vi "PH_AWG-510.PC Write PSDB.vi"(0 "i ref in":refnum<vi>, 5 "error IO":errorcluster) -> (14 "i ref out":refnum<vi>, 19 "error out":errorcluster)   [LabVIEW 2014, in "PH_AWG-510.lvlib"]
doc: "This is the proc case which writes data to the PHELIX shot data base."
uses:
  PH_AWG-510.lvlib
  PH_Basics/PH_PSDBWriter/PH_PSDBWriter.PSDB Dataset.ctl
  PH_Basics/PH_PSDBWriter/PH_PSDBWriter.2D dataset.ctl
  CSlibraries-extern/psdb_lv/PSDB_AxisDescription.ctl
  PH_Basics/PH_PSDBWriter/PH_PSDBWriter.Boolean dataset.ctl
  PH_Basics/PH_PSDBWriter/PH_PSDBWriter.Image dataset.ctl
  <vilib>/vision/Image Controls.llb/IMAQ Image.ctl
  PH_Basics/PH_PSDBWriter/PH_PSDBWriter.Numeric dataset.ctl
  PH_Basics/PH_PSDBWriter/PH_PSDBWriter.String dataset.ctl
  PH_Basics/PH_PSDBWriter/PH_PSDBWriter.lvlib
  CSlibraries-extern/psdb_lv/PSDB.lvlib
  PH_Basics/PH_StatusHandler/PH_StatusHandler.lvlib
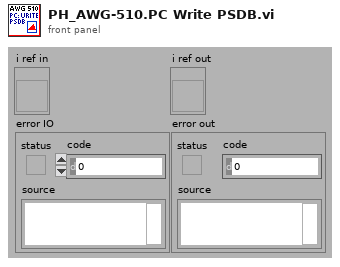
[diagram p1: front panel]
types:
  T1 = typedef "PH_PSDBWriter.lvlib/PH_PSDBWriter.PSDB Dataset.ctl" = cluster{"Version":i32, "2D data Input":T2[], "Boolean Input":T4[], "Image Input":T5[], "Numeric Input":T7[], "String Input":T8[]}
  T2 = typedef "PH_PSDBWriter.lvlib/PH_PSDBWriter.2D dataset.ctl" = cluster{"name":string, "data":dbl[][], "axis description":T3}
  T3 = typedef "PSDB.lvlib/PSDB_AxisDescription.ctl" = cluster{"x axis label":string, "y axis label":string, "x axis unit":string, "y axis unit":string}
  T4 = typedef "PH_PSDBWriter.lvlib/PH_PSDBWriter.Boolean dataset.ctl" = cluster{"name":string, "data":bool, "unit":string}
  T5 = typedef "PH_PSDBWriter.lvlib/PH_PSDBWriter.Image dataset.ctl" = cluster{"name":string, "data":T6, "unit":string}
  T6 = typedef "IMAQ Image.ctl" = refnum<image>
  T7 = typedef "PH_PSDBWriter.lvlib/PH_PSDBWriter.Numeric dataset.ctl" = cluster{"name":string, "data":dbl, "unit":string}
  T8 = typedef "PH_PSDBWriter.lvlib/PH_PSDBWriter.String dataset.ctl" = cluster{"name":string, "data":string, "unit":string}
  T9 = typedef "PH_AWG-510.lvlib/PH_AWG-510.i attribute.ctl" = cluster{"GUI Refs":cluster{"Delete":refnum<vi>, "Trigger Settings":refnum<vi>, "Start Device":refnum<vi>, "Instrument Information":refnum<vi>, "Lock Frontpanel":refnum<vi>, "Waveform Pattern File":refnum<vi>, "Initialize":refnum<vi>, "Output Settings":refnum<vi>}, "Instrument Information":T10, "Initialized?":bool, "Current Settings":cluster{"Trigger":T11, "Output Settings":T12}, "Wanted Settings":cluster{"Trigger":T11, "Output Settings":T12}, "Device frontpanel locked?":bool, "Default File Path":path}
  T10 = typedef "PH_AWG-510.lvlib/PH_AWG-510.Instrument Information Dataset.ctl" = cluster{"VISA resource name":refnum<visa-resource-name>, "Instrument Firmware Revision":string, "Manufacturer":string, "Model":string, "Serial Number":string, "Error Message":string, "Device Status":enum16{"stopped", "wating for trigger", "running", "Failure"}}
  T11 = typedef "PH_AWG-510.lvlib/PH_AWG-510.Trigger Settings.ctl" = cluster{"Mode":enum16{"Continuous", "Triggered", "Gated", "Enhanced"}, "Level (V)":dbl, "External Source":bool}
  T12 = typedef "PH_AWG-510.lvlib/PH_AWG-510.Output Settings.ctl" = cluster{"Activate Channel":bool, "VPP (V)":dbl, "Clock (Hz)":dbl, "File Name (Device)":string, "#1":u16, "#2":u16, "#3":u16, "#4":u16, "#5":u16, "#6":u16, "#7":u16, "#8":u16, "#9":u16, "#10":u16, "#11":u16, "#12":u16, "#13":u16, "#14":u16, "#15":u16, "#16":u16, "#17":u16, "#18":u16, "#19":u16, "#20":u16, "Offset (V)":dbl}
  T13 = typedef "PH_StatusHandler.lvlib/PH_StatusHandler.Status.ctl" = i16
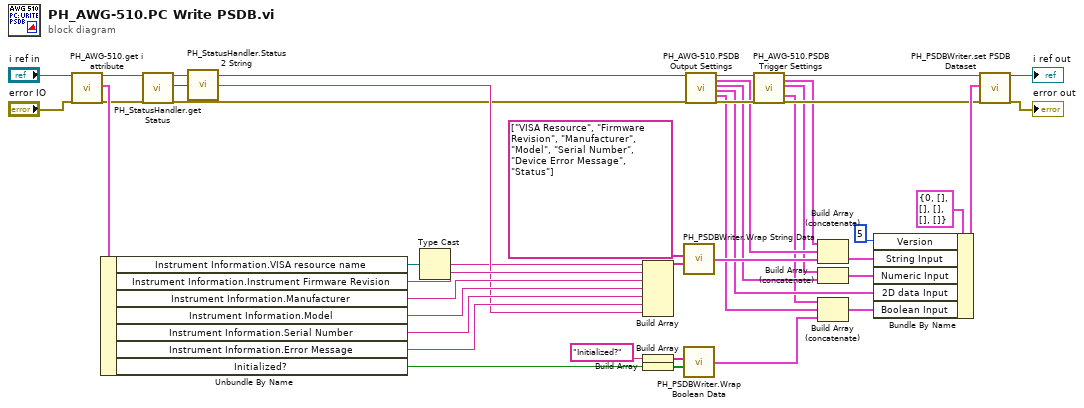
[diagram p0: block diagram]
diagram:
  n1 = call "PH_AWG-510.get i attribute.vi"("i ref in"="i ref in", "error in (no error)"="error IO") -> ("i ref out"=w3:refnum<vi>, "i attribute"=w38:T9, "error out"=w19:errorcluster)  [unwired: 15 in]
  n2 = Unbundle By Name(w38) -> ("Instrument Information.VISA resource name"=w28:refnum<visa-resource-name>, "Instrument Information.Instrument Firmware Revision"=w37:string, "Instrument Information.Manufacturer"=w36:string, "Instrument Information.Model"=w35:string, "Instrument Information.Serial Number"=w34:string, "Instrument Information.Error Message"=w33:string, "Initialized?"=w23:bool)
  n3 = call "PH_StatusHandler.get Status.vi"("VI in"=w3, "error in"=w19) -> ("VI out"=w2:refnum<vi>, "Status"=w1:T13, "error out"=w4:errorcluster)  [unwired: 15 in]
  n4 = call "PH_StatusHandler.Status 2 String.vi"("Status"=w1) -> ("Status as string"=w32:string)
  n5 = Type Cast(x=w28) -> (*(type *) &x=w27:string)  [unwired: 1 in]
  n6 = Build Array(w27, w37, w36, w35, w34, w33, w32) -> (w29:string[])
  n7 = Build Array("Initialized?") -> (w24:string[])
  n8 = Build Array(w23) -> (w25:bool[])
  n9 = call "PH_PSDBWriter.Wrap String Data.vi"("Data Array"=w29, "Name Array"=string[] ["VISA Resource", "Firmware Revision", "Manufacturer", "Model", "Serial Number", "Device Error Message", "Status"]) -> ("PSDB String Data Array"=w26:T8[])  [unwired: 2 in]
  n10 = call "PH_PSDBWriter.Wrap Boolean Data.vi"("Data Array"=w25, "Name Array"=w24) -> ("PSDB Boolean Data Array"=w6:T4[])  [unwired: 2 in]
  n11 = call "PH_AWG-510.PSDB Output Settings.vi"("i ref in"=w2, "error IO"=w4) -> ("i ref out"=w17:refnum<vi>, "Output Settings PSDB String Data"=w14:T8[], "Output Settings PSDB Numeric Data"=w12:T7[], "Output Settings PSDB 2D Data"=w9:T2[], "Output Settings PSDB Boolean Data"=w7:T4[], "error out"=w20:errorcluster)  [unwired: 12 in]
  n12 = call "PH_AWG-510.PSDB Trigger Settings.vi"("i ref in"=w17, "error IO"=w20) -> ("i ref out"=w16:refnum<vi>, "Trigger Settings PSDB String Data"=w13:T8[], "Trigger Settings PSDB Numeric Data"=w11:T7[], "Trigger Settings PSDB Boolean Data"=w8:T4[], "error out"=w18:errorcluster)  [unwired: 13 in]
  n13 = Build Array (concatenate)(w13, w14, w26) -> (w15:T8[])
  n14 = Build Array (concatenate)(w11, w12) -> (w10:T7[])
  n15 = Build Array (concatenate)(w8, w7, w6) -> (w5:T4[])
  n16 = Bundle By Name(cluster=T1 {"Version"=0, "2D data Input"=[], "Boolean Input"=[], "Image Input"=[], "Numeric Input"=[], "String Input"=[]} ("PSDB Dataset"), "Version"=5, "String Input"=w15, "Numeric Input"=w10, "2D data Input"=w9, "Boolean Input"=w5) -> (w31:T1)
  n17 = call "PH_PSDBWriter.set PSDB Dataset.vi"("VI in"=w16, "PSDB Dataset"=w31, "error in (no error)"=w18) -> ("VI out"=→"i ref out":refnum<vi>, "error out"=→"error out":errorcluster)  [unwired: 15 in]
